vi "prima_apl_v4.vi"() -> ()   [LabVIEW 2009]
panel:
  out "Terminal de tip Numeric":dbl
  # "Aplicatia afiseaza valoarea lui pi"
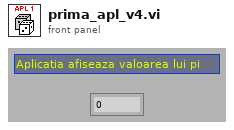
[diagram p1: front panel]
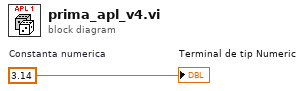
[diagram p0: block diagram]
diagram:
  w1 = 3.14  # Constanta numerica
  "Terminal de tip Numeric" <- w1
